vi "DAQ.Read.vi"(8 "error in (no error)":errorcluster, 11 "DAQmx.AI in":refnum<class "DAQmx.AI.lvclass">) -> (0 "error out":errorcluster, 2 "Read":waveform(dbl)[](array[waveform]), 3 "DAQmx.AI out":refnum<class "DAQmx.AI.lvclass">)   [LabVIEW 2016, in "DAQmx.AI.lvclass"]
uses:
  DAQmx.AI.lvclass
  C:/user/patrick/hg/levy_inst_lockin.SMO/lvsrc/SMOs/DAQmx/DAQmx.lvclass
  C:/user/patrick/hg/levy_inst_lockin.SMO/lvsrc/SMOs/DAQ/DAQ.lvclass
  DAQmx/DAQmx.lvclass/DAQmx.ctl
  DAQ/DAQ.lvclass/DAQ.ctl
  <vilib>/DAQmx/read.llb/DAQmx Read (Analog 1D Wfm NChan NSamp).vi
  <vilib>/DAQmx/miscellaneous.llb/DAQmx Fill In Error Info.vi
  DAQ/DAQ.lvclass
  <resource>/objmgr/daqmx.rc
  DAQmx/DAQmx.lvclass
panel:
  out "AvailSampPerChan":u32
  out "Numeric":i32
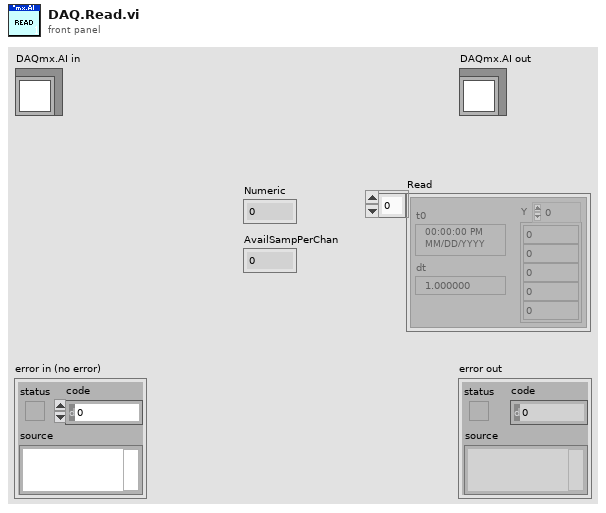
[diagram p1: front panel]
types:
  T1 = typedef "DAQ.lvclass/DAQ_Config.ctl" = cluster{"Channels":T2, "DAQ_Type":T3, "minimum value":dbl, "maximum value":dbl, "DAQ_SamplingInfo":T4, "DAQ_SamplingMode":T5}
  T2 = typedef "DAQ.lvclass/PrivateEvents--DAQ.AI.Channels.ctl" = string
  T3 = typedef "DAQ.lvclass/DAQ_Type.ctl" = enum16{"AI", "AO"}
  T4 = typedef "DAQ.lvclass/DAQ_SamplingInfo.ctl" = cluster{"Fs":dbl, "#s":i32}
  T5 = typedef "DAQ.lvclass/DAQ_SamplingMode.ctl" = enum16{"Continuous", "Finite"}
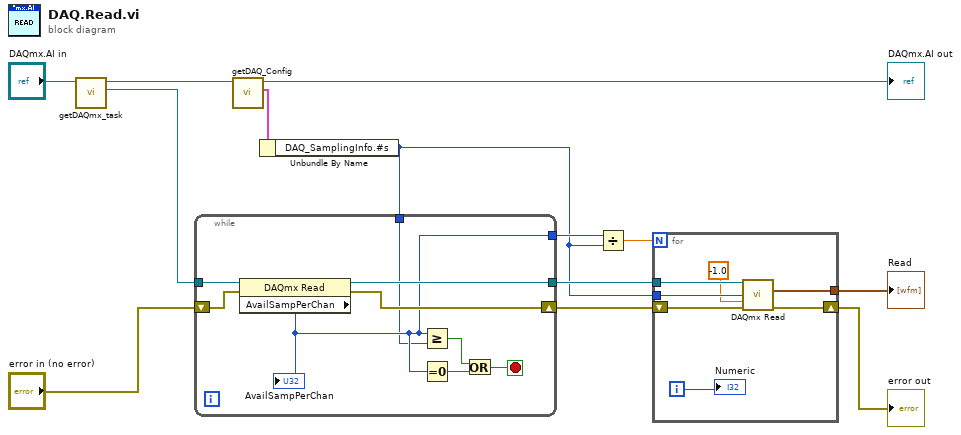
[diagram p0: block diagram]
diagram:
  n1 = call "getDAQmx_task.vi"("DAQmx in"="DAQmx.AI in") -> ("task"=w4:refnum<k21>, "DAQmx out"=w3:refnum<class "DAQmx.AI.lvclass">)  [unwired: 8 in, 1 out]
  n2 = call "getDAQ_Config.vi"("DAQ in"=w3) -> ("DAQ_Config"=w8:T1, "DAQ out"=→"DAQmx.AI out":refnum<class "DAQmx.AI.lvclass">)  [unwired: 8 in, 1 out]
  n3 = Unbundle By Name(w8) -> ("DAQ_SamplingInfo.#s"=w5:i32)
  n4 = while {
    tunnel: [w22] -> w12
    tunnel: [w16] -> w6
    tunnel: w4 -> [w17]
    shift-right: [w21] -> w13
    shift-left: "error in (no error)" -> [w15]
    tunnel: w5 -> [w14]
    stop <- w20 stop-if-true
    n5 = property class="DAQmx Read"(reference=w17, error in=w15) -> (reference out=w22:refnum<k21>, error out=w21:errorcluster, "AvailSampPerChan"=w16:u32)
    "AvailSampPerChan" <- w16
    n6 = Greater Or Equal?(x=w16, y=w14) -> (x >= y?=w18:bool)
    n7 = Equal To 0?(x=w16) -> (x = 0?=w19:bool)
    n8 = Or(x=w18, y=w19) -> (x .or. y?=w20:bool)
  }
  n9 = Divide(x=w6, y=w5) -> (x/y=w7:dbl)
  n10 = for {
    N: w7 -> [_]
    tunnel: w12 -> [w29]
    tunnel: [w28] -> w9
    tunnel: w5 -> [w27]
    shift-right: [w26] -> w10
    shift-left: w13 -> [w23]
    i -> [w25]
    n11 = call-poly <vilib>:"DAQmx Read.vi"("task/channels in"=w29, "number of samples per channel"=w27, "timeout"=-1.0, "error in"=w23) -> ("data"=w28:waveform(dbl)[], "error out"=w26:errorcluster)  [unwired: 9 in, 1 out]
    "Numeric" <- w25
  }
  "error out" <- w10
  "Read" <- w9
